vi "Get Video Stream(SubVI).vi"() -> (0 "error out":errorcluster, 3 "ImgData":u8[](array[numeric]))   [LabVIEW 2014]
uses:
  <vilib>/LVH/AR Drone Toolkit/Decode Video/2.0/Decode20Video.dll
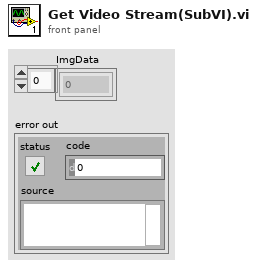
[diagram p1: front panel]
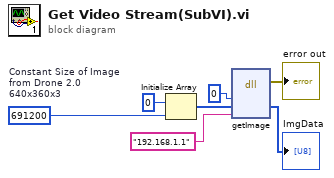
[diagram p0: block diagram]
diagram:
  w1 = 691200  # Constant Size of Image from Drone 2.0 640x360x3
  n1 = Initialize Array(u8 0 ("dimension size"), w1) -> (w3:u8[])
  n2 = dll-call lib="C:/Program Files (x86)/National Instruments/LabVIEW 2014/vi.lib/LVH/AR Drone Toolkit/Decode Video/2.0/Decode20Video.dll" fn="getImage"("Index"=0, "ImgData"=w3, "IP Address"="192.168.1.1") -> (error out=→"error out":errorcluster, "ImgData"=→"ImgData":u8[])  [unwired: 6 in, 1 out]
